vi "LabvolutionSubmoduleCheck_FormatPath.vi"(11 "Path in":path) -> (3 "String out":string)   [LabVIEW 2018]
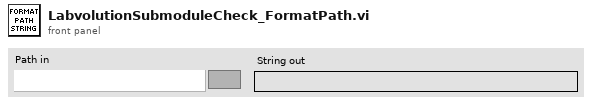
[diagram p1: front panel]
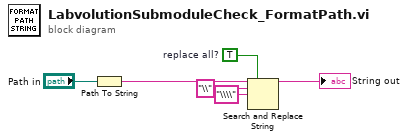
[diagram p0: block diagram]
diagram:
  w3 = TRUE  # replace all?
  n1 = Path To String(path="Path in") -> (string=w2:string)
  n2 = Search and Replace String(replace all?=w3, input string=w2, search string="\\", replace string="\\\\" ("replace string (\"\")")) -> (result string=→"String out":string)  [unwired: 4 in, 3 out]
